vi "BRig_RT_comm_webdav_upload__gatherFilenames__v3.vi"() -> (2 "output_arrBlank":bool[](array[boolean]), 3 "output_arrFilenames":string[](array[string]), 5 "output_n":i32)   [LabVIEW 2014]
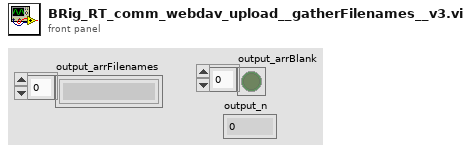
[diagram p1: front panel]
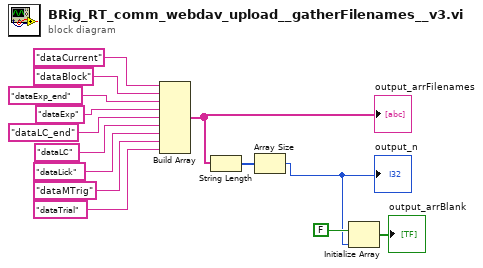
[diagram p0: block diagram]
diagram:
  n1 = Build Array("dataCurrent" ("input_filename"), "dataBlock" ("input_filename"), "dataExp_end" ("input_filename"), "dataExp" ("input_filename"), "dataLC_end" ("input_filename"), "dataLC" ("input_filename"), "dataLick" ("input_filename"), "dataMTrig" ("input_filename"), "dataTrial" ("input_filename")) -> (w10:string[])
  "output_arrFilenames" <- w10
  n2 = String Length(string=w10) -> (length=w9:i32[])
  n3 = Array Size(array=w9) -> (size(s)=w8:i32)
  "output_n" <- w8
  n4 = Initialize Array(FALSE, w8) -> (→"output_arrBlank":bool[])
